vi "Write AIs RT FIFO.vi"(8 "error in (no error)":errorcluster, 10 "AI Values":sgl[](array[numeric]), 11 "AIs RT FIFO out":refnum<k33>) -> (0 "error out":errorcluster)   [LabVIEW 2021, in "RT Main.lvlib"]
uses:
  RT Main.lvlib
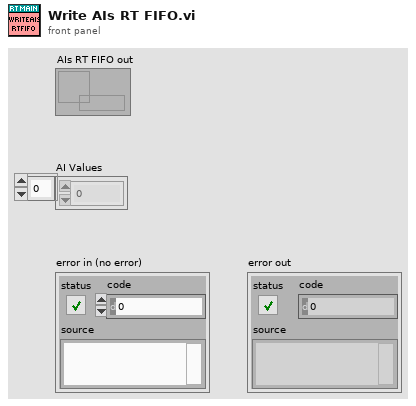
[diagram p1: front panel]
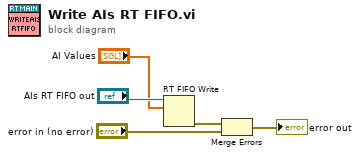
[diagram p0: block diagram]
diagram:
  n1 = RT FIFO Write(0:"AIs RT FIFO out", 1:"AI Values") -> (11:w3:errorcluster)  [unwired: 3 in, 3 out]
  n2 = Merge Errors(w3, "error in (no error)") -> (→"error out":errorcluster)
